vi "Sistema de ventilación_V4.vi"() -> ()   [LabVIEW 2023]
uses:
  <vilib>/MakerHub/LINX/Public/Peripherals/Analog/Analog Read 1 Chan.vi
  <vilib>/MakerHub/LINX/Public/Peripherals/Digital/Digital Write 1 Chan.vi
  <vilib>/MakerHub/LINX/Public/Peripherals/Analog/Analog Read N Chans.vi
  <vilib>/MakerHub/LINX/Public/Peripherals/Digital/Digital Write N Chans.vi
  <vilib>/MakerHub/LINX/Private/Local IO/LinxAnalogRead.vi
  <vilib>/MakerHub/LINX/Public/Utilities/Check Channel.vi
  <vilib>/MakerHub/LINX/Private/Local IO/LinxDigitalWrite.vi
  <vilib>/MakerHub/LINX/Public/Utilities/Open Serial.vi
  <vilib>/MakerHub/LINX/Public/Sensors/Motion/Servo/Servo Open One Channel.vi
  <vilib>/MakerHub/LINX/Public/Peripherals/Analog/Analog Write 1 Chan.vi
  <vilib>/MakerHub/LINX/Private/Utilties/Generate Error.vi
  <vilib>/MakerHub/LINX/Public/Sensors/Motion/Servo/Servo Set Pulse Width One Channel.vi
  <vilib>/MakerHub/LINX/Public/Sensors/Motion/Servo/Servo Close One Channel.vi
  <vilib>/MakerHub/LINX/LMH-LINX.lvlib
  <vilib>/MakerHub/LINX/Public/Sensors/Motion/Servo/Servo.lvlib
panel:
  in  "Temp":dbl(knob) scale=-20.0..100.0
  in  "Aire":dbl(knob) scale=0.0..1000.0
  out "?":bool
  out "?":bool
  out "?":bool
  out "?":bool
  in  "?":bool
  out "Serevo Aire Angulo":string
  out "Serevo Temp Angulo":string
  in  "Serial Port":refnum<visa-resource-name>
  out "?":bool
  out "?":bool
  out "?":bool
  out "?":bool
  out "?":bool
  out "?":bool
  out "?":bool
  out "?":bool
  out "?":bool
  out "?":bool
  out "?":bool
  out "?":bool
  out "?":bool
  out "?":bool
  out "?":bool
  out "?":bool
  out "?":bool
  out "?":bool
  in  "?":bool
  out "Filtro de Calor":bool
  out "Filtro de Aire":bool
  out "Ppm del aire":dbl(knob) scale=0.0..1800.0
  out "Temperatura":dbl(slide) scale=0.0..60.0
  out "t [sec]":dbl
  out "Iteration No":i32
  in  "?":bool
  out "VI is running?":bool caption="ON/OFF"
  # "SISTEMA DE VENTILACIÓN DE DOBLE FLUJO"
  # "Temperatura"
  # "Entrada"
  # "Calidad del aire"
  # "Salida"
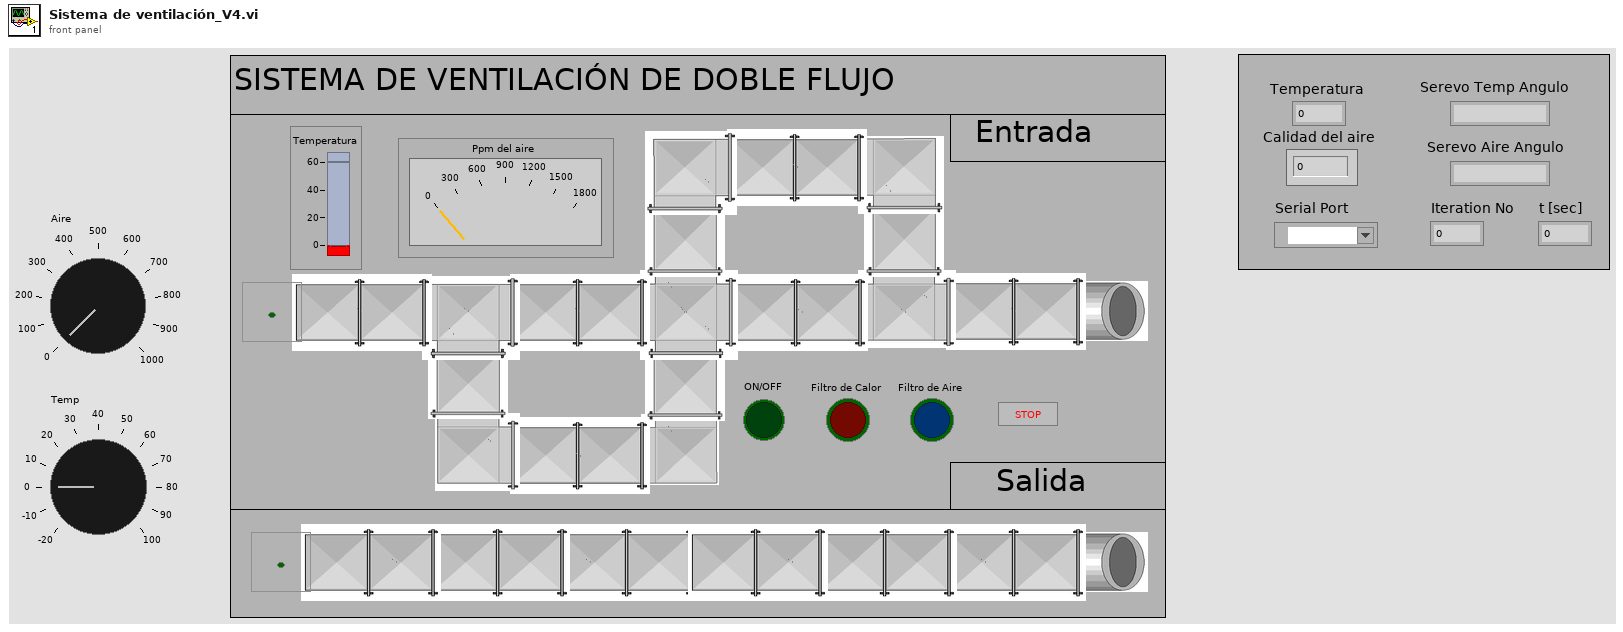
[diagram p1: front panel]
types:
  T1 = typedef "LMH-LINX.lvlib/LINX Ref.ctl" = cluster{"IO":T2, "Interface":T3, "LINX Device Config":T4}
  T2 = typedef "LMH-LINX.lvlib/Platform.ctl" = enum16{"Remote", "Local"}
  T3 = typedef "LMH-LINX.lvlib/Interface.ctl" = enum16{"Serial", "TCP"}
  T4 = typedef "LMH-LINX.lvlib/Device.lvlib/LINX Device Config.ctl" = cluster{"Interface":T3, "COM Port":refnum<visa-resource-name>, "TCP Configuration":T5, "Device Family":u8, "Device ID":u8, "Device Name":string, "TCP Ref":refnum<k5>, "Channels":T6}
  T5 = typedef "LMH-LINX.lvlib/Device.lvlib/TCP Config.ctl" = cluster{"IP Address":string, "Port":u16}
  T6 = typedef "LMH-LINX.lvlib/Channels.ctl" = cluster{"DI":u8[], "DO":u8[], "AI":u8[], "AO":u8[], "PWM":u8[], "QE":u8[], "UART":u8[], "I2C 2":u8[], "SPI":u8[], "CAN":u8[], "Servo":u8[], "AI Ref (V)":dbl, "AI Resolution (Bits)":u8, "AO Ref (V)":dbl, "AO Resolution (Bits)":u8}
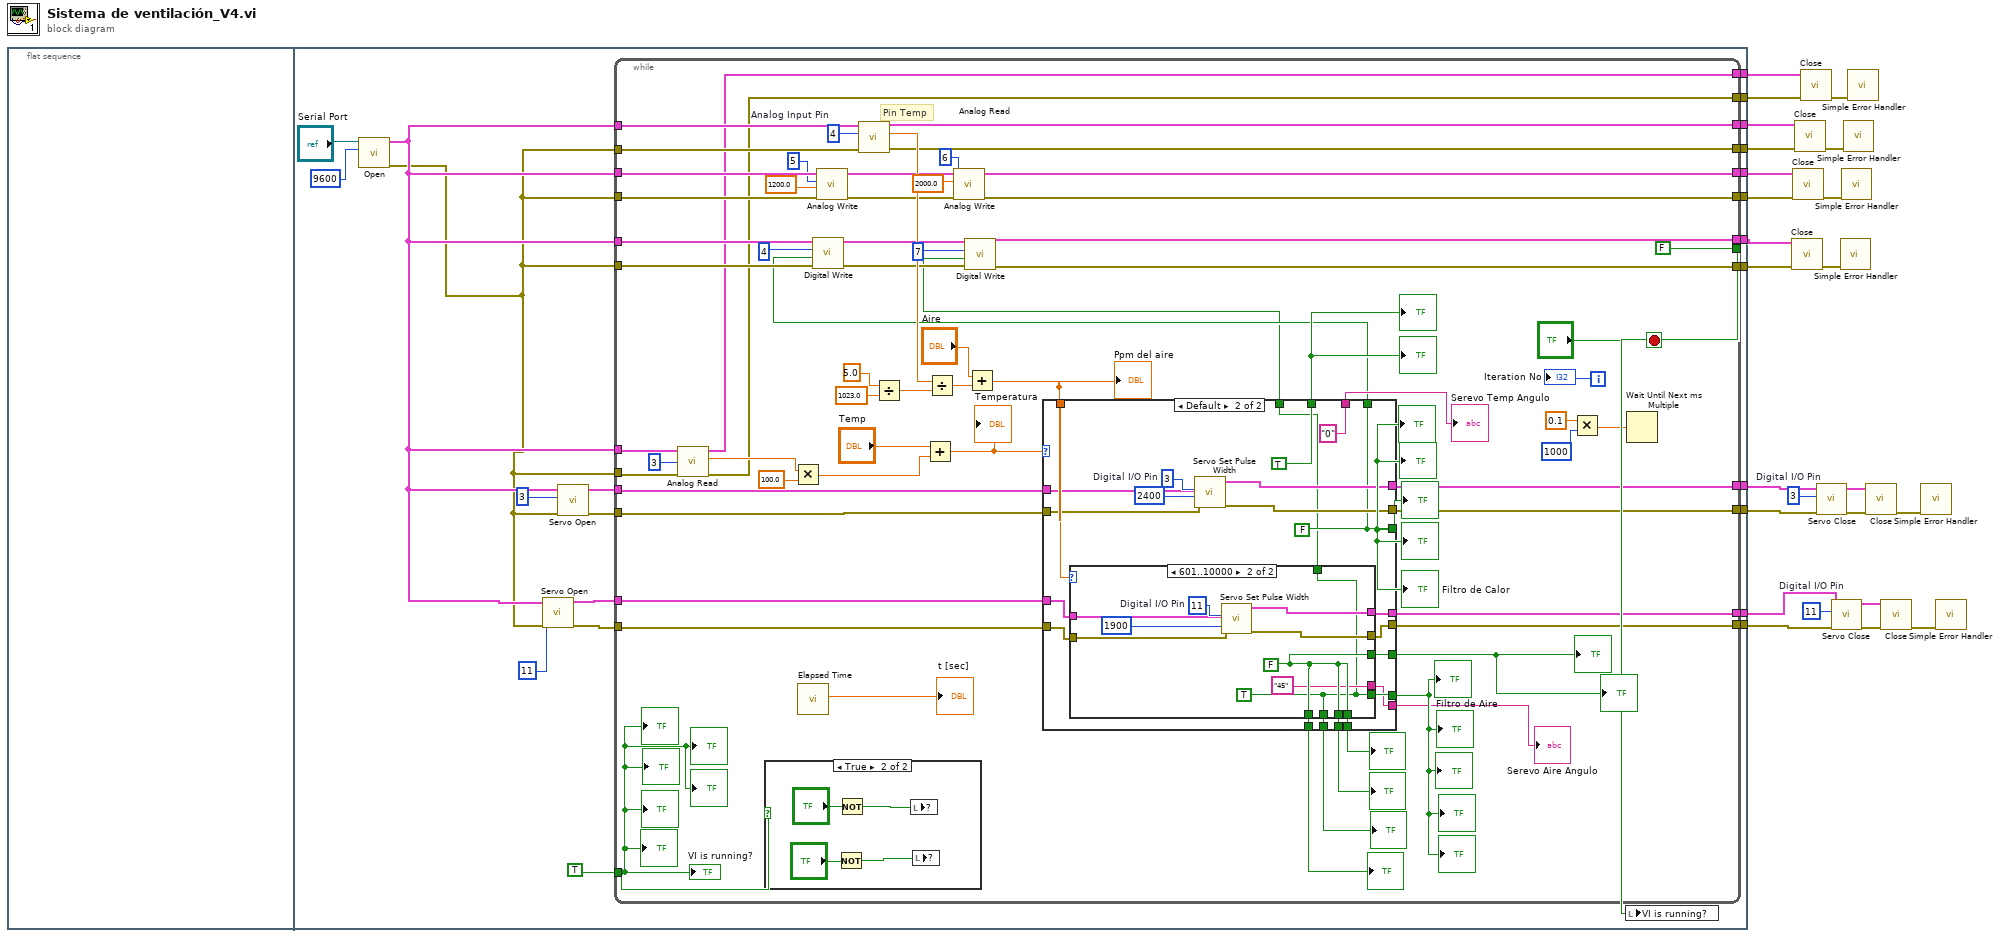
[diagram p0: block diagram]
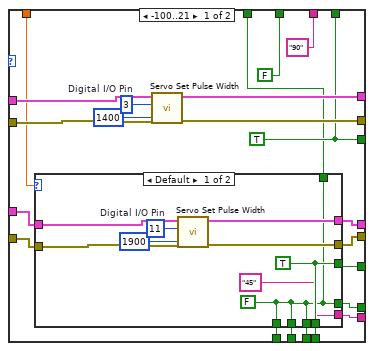
[diagram p2: hidden frame]
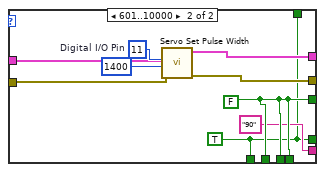
[diagram p3: hidden frame]
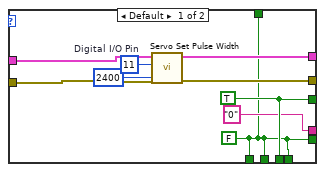
[diagram p4: hidden frame]
diagram:
  w7 = 11  # Digital I/O Pin
  w13 = 3  # Digital I/O Pin
  n1 = flat-sequence {
    tunnel: [w45] -> w24
    tunnel: [w43] -> w22
    tunnel: [w42] -> w20
    tunnel: [w41] -> w19
    tunnel: [w40] -> w17
    tunnel: [w39] -> w16
    tunnel: [w38] -> w1
    tunnel: [w37] -> w14
    tunnel: [w34] -> w9
    tunnel: [w33] -> w8
    tunnel: [w32] -> w3
    tunnel: [w31] -> w2
    frame #0 {
    }
    frame #1 {
      n2 = call-poly <vilib>:"Open.vi"("Baud Rate Override"=u32 9600, "Serial Port"="Serial Port") -> ("Error Out"=w27:errorcluster, "LINX Resource"=w29:T1)  [unwired: 7 in, 1 out]
      n3 = call-poly <vilib>:"Servo Open.vi"("Error In"=w27, "Servo Channel"=u8 11, "LINX Resource"=w29) -> ("Error Out"=w26:errorcluster, "LINX Resource"=w28:T1)  [unwired: 7 in]
      n4 = call-poly <vilib>:"Servo Open.vi"("Error In"=w27, "Servo Channel"=u8 3, "LINX Resource"=w29) -> ("Error Out"=w35:errorcluster, "LINX Resource"=w36:T1)  [unwired: 7 in]
      n5 = while {
        tunnel: [FALSE] -> w47
        tunnel: TRUE -> [w90]
        tunnel: w29 -> [w53]
        tunnel: [w55] -> w45
        tunnel: w27 -> [w52]
        tunnel: w29 -> [w109]
        tunnel: [w54] -> w43
        tunnel: w27 -> [w104]
        tunnel: [w102] -> w42
        tunnel: [w101] -> w41
        tunnel: w27 -> [w100]
        tunnel: w29 -> [w99]
        tunnel: [w92] -> w40
        tunnel: [w91] -> w39
        tunnel: w27 -> [w89]
        tunnel: w29 -> [w88]
        tunnel: [w83] -> w38
        tunnel: [w82] -> w37
        tunnel: w36 -> [w81]
        tunnel: w35 -> [w80]
        tunnel: [w79] -> w34
        tunnel: [w78] -> w33
        tunnel: w28 -> [w72]
        tunnel: w26 -> [w71]
        tunnel: [w70] -> w32
        tunnel: [w69] -> w31
        i -> [w111]
        stop <- "?" stop-if-true
        w103 = 4  # Analog Input Pin
        # "Pin Temp"
        n6 = call-poly <vilib>:"Analog Read.vi"("Error In"=w52, "Analog Channel"=u8 3, "LINX Resource"=w53) -> ("Error Out"=w54:errorcluster, "Voltage"=w57:dbl, "LINX Resource"=w55:T1)  [unwired: 5 in, 1 out]
        n7 = case shown="True" w90 {
          frame False {
          }
          frame True {
            n8 = Not(x="?") -> (.not. x?=w197:bool)
            n9 = Not(x="?") -> (.not. x?=w199:bool)
            n10 = local write item#8(w199) -> ()
            n11 = local write item#30(w197) -> ()
          }
        }
        n12 = Multiply(x=w57, y=100.0 ("x")) -> (x*y=w56:dbl)
        n13 = call "Elapsed Time"() -> ("Elapsed Time (s)"=→"t [sec]":dbl)  [unwired: 12 in, 7 out]
        n14 = call-poly <vilib>:"Analog Write.vi"("Error In"=w100, "AO Value"=1200.0, "AO Channel"=5, "LINX Resource"=w99) -> ("Error Out"=w93:errorcluster, "LINX Resource"=w94:T1)  [unwired: 6 in]
        n15 = call-poly <vilib>:"Analog Read.vi"("Error In"=w104, "Analog Channel"=w103, "LINX Resource"=w109) -> ("Error Out"=w101:errorcluster, "Voltage"=w106:dbl, "LINX Resource"=w102:T1)  [unwired: 5 in, 1 out]
        n16 = Divide(x=5.0, y=1023.0) -> (x/y=w105:dbl)
        n17 = Add(x="Temp", y=w56) -> (x+y=w74:dbl)
        "Temperatura" <- w74
        n18 = Divide(x=w106, y=w105) -> (x/y=w76:dbl)
        n19 = call-poly <vilib>:"Analog Write.vi"("Error In"=w93, "AO Value"=2000.0, "AO Channel"=6, "LINX Resource"=w94) -> ("Error Out"=w92:errorcluster, "LINX Resource"=w91:T1)  [unwired: 6 in]
        n20 = Add(x="Aire", y=w76) -> (x+y=w68:dbl)
        "Ppm del aire" <- w68
        n21 = case shown="Default" w74 {
          tunnel: w81 -> [w136 w176]
          tunnel: w80 -> [w135 w175]
          tunnel: [w134 w174] -> w79
          tunnel: [w133 w173] -> w78
          tunnel: [w118 w158] -> w73
          tunnel: [FALSE TRUE] -> w51
          tunnel: w72 -> [w128 w166]
          tunnel: w71 -> [w127 w165]
          tunnel: [w125 w167] -> w70
          tunnel: [w126 w168] -> w69
          tunnel: w68 -> [w129 w169]
          tunnel: [w131 w171] -> w67
          tunnel: [w130 w170] -> w66
          tunnel: [w124 w164] -> w65
          tunnel: [w121 w163] -> w64
          tunnel: [w122 w162] -> w63
          tunnel: [w123 w161] -> w62
          tunnel: ["90" ("Serevo Temp Angulo") "0" ("Serevo Temp Angulo")] -> w61
          tunnel: [w119 w159] -> w60
          tunnel: [w118 w158] -> w50
          tunnel: [w117 w157] -> w49
          frame -100..21 {
            w118 = TRUE
            w138 = 3  # Digital I/O Pin
            n22 = case shown="Default" w129 {
              tunnel: w128 -> [w145 w154]
              tunnel: w127 -> [w144 w153]
              tunnel: [w143 w152] -> w126
              tunnel: [w142 w151] -> w125
              tunnel: [w141 w150] -> w131
              tunnel: [w139 w148] -> w130
              tunnel: [w141 w150] -> w124
              tunnel: [w139 w148] -> w123
              tunnel: [w139 w150] -> w122
              tunnel: [w139 w150] -> w121
              tunnel: ["45" ("Serevo Aire Angulo") "90" ("Serevo Aire Angulo")] -> w119
              tunnel: [w139 w148] -> w117
              frame Default {
                w139 = FALSE
                w141 = TRUE
                w147 = 11  # Digital I/O Pin
                n23 = call-poly <vilib>:"Servo Set Pulse Width.vi"("Error In"=w144, "Pulse Width (uS)"=u16 1900, "Servo Channel"=w147, "LINX Resource"=w145) -> ("Error Out"=w142:errorcluster, "LINX Resource"=w143:T1)  [unwired: 6 in]
              }
              frame 601..10000 {
                w150 = FALSE
                w148 = TRUE
                w156 = 11  # Digital I/O Pin
                n24 = call-poly <vilib>:"Servo Set Pulse Width.vi"("Error In"=w153, "Pulse Width (uS)"=u16 1400, "Servo Channel"=w156, "LINX Resource"=w154) -> ("Error Out"=w151:errorcluster, "LINX Resource"=w152:T1)  [unwired: 6 in]
              }
            }
            n25 = call-poly <vilib>:"Servo Set Pulse Width.vi"("Error In"=w135, "Pulse Width (uS)"=u16 1400, "Servo Channel"=w138, "LINX Resource"=w136) -> ("Error Out"=w133:errorcluster, "LINX Resource"=w134:T1)  [unwired: 6 in]
          }
          frame Default {
            w158 = FALSE
            w178 = 3  # Digital I/O Pin
            n26 = case shown="601..10000" w169 {
              tunnel: w166 -> [w185 w195]
              tunnel: w165 -> [w184 w194]
              tunnel: [w183 w193] -> w168
              tunnel: [w182 w192] -> w167
              tunnel: [w181 w191] -> w171
              tunnel: [w179 w189] -> w170
              tunnel: [w179 w191] -> w164
              tunnel: [w181 w191] -> w163
              tunnel: [w179 w189] -> w162
              tunnel: [w179 w191] -> w161
              tunnel: ["0" ("Serevo Aire Angulo") "45" ("Serevo Aire Angulo")] -> w159
              tunnel: [w179 w189] -> w157
              frame Default {
                w179 = FALSE
                w181 = TRUE
                w187 = 11  # Digital I/O Pin
                n27 = call-poly <vilib>:"Servo Set Pulse Width.vi"("Error In"=w184, "Pulse Width (uS)"=u16 2400, "Servo Channel"=w187, "LINX Resource"=w185) -> ("Error Out"=w182:errorcluster, "LINX Resource"=w183:T1)  [unwired: 6 in]
              }
              frame 601..10000 {
                w191 = FALSE
                w189 = TRUE
                w196 = 11  # Digital I/O Pin
                n28 = call-poly <vilib>:"Servo Set Pulse Width.vi"("Error In"=w194, "Pulse Width (uS)"=u16 1900, "Servo Channel"=w196, "LINX Resource"=w195) -> ("Error Out"=w192:errorcluster, "LINX Resource"=w193:T1)  [unwired: 6 in]
              }
            }
            n29 = call-poly <vilib>:"Servo Set Pulse Width.vi"("Error In"=w175, "Pulse Width (uS)"=u16 2400, "Servo Channel"=w178, "LINX Resource"=w176) -> ("Error Out"=w173:errorcluster, "LINX Resource"=w174:T1)  [unwired: 6 in]
          }
        }
        "?" <- w63
        "?" <- w64
        "?" <- w62
        "?" <- w65
        "Serevo Temp Angulo" <- w61
        "Serevo Aire Angulo" <- w60
        "?" <- w73
        "?" <- w73
        "?" <- w73
        "?" <- w73
        "Filtro de Calor" <- w73
        "?" <- w51
        "?" <- w51
        "Filtro de Aire" <- w66
        "?" <- w66
        "?" <- w66
        "?" <- w66
        "?" <- w66
        "?" <- w67
        "?" <- w67
        n30 = call-poly <vilib>:"Digital Write.vi"("Error In"=w89, "Output Value"=w50, "DO Channel"=4, "LINX Resource"=w88) -> ("Error Out"=w84:errorcluster, "LINX Resource"=w85:T1)  [unwired: 6 in]
        n31 = call-poly <vilib>:"Digital Write.vi"("Error In"=w84, "Output Value"=w49, "DO Channel"=7, "LINX Resource"=w85) -> ("Error Out"=w82:errorcluster, "LINX Resource"=w83:T1)  [unwired: 6 in]
        n32 = Multiply(x=0.1, y=1000) -> (x*y=w114:dbl)
        n33 = Wait Until Next ms Multiple(millisecond multiple=w114) -> ()  [unwired: 1 out]
        "VI is running?" <- w90
        "Iteration No" <- w111
        "?" <- w90
        "?" <- w90
        "?" <- w90
        "?" <- w90
        "?" <- w90
        "?" <- w90
      }
      n34 = local write "VI is running?"(w47) -> ()
    }
  }
  n35 = call <vilib>:"Close.vi"("Error In"=w14, "LINX Resource"=w1) -> ("Error Out"=w15:errorcluster)  [unwired: 9 in]
  n36 = call <vilib>:"Close.vi"("Error In"=w17, "LINX Resource"=w16) -> ("Error Out"=w18:errorcluster)  [unwired: 9 in]
  n37 = call <vilib>:"Close.vi"("Error In"=w19, "LINX Resource"=w20) -> ("Error Out"=w21:errorcluster)  [unwired: 9 in]
  n38 = call <vilib>:"Close.vi"("Error In"=w22, "LINX Resource"=w24) -> ("Error Out"=w23:errorcluster)  [unwired: 9 in]
  n39 = call-poly <vilib>:"Servo Close.vi"("Error In"=w8, "Servo Channel"=w13, "LINX Resource"=w9) -> ("Error Out"=w11:errorcluster, "LINX Resource"=w12:T1)  [unwired: 7 in]
  n40 = call-poly <vilib>:"Servo Close.vi"("Error In"=w3, "Servo Channel"=w7, "LINX Resource"=w2) -> ("Error Out"=w5:errorcluster, "LINX Resource"=w6:T1)  [unwired: 7 in]
  n41 = call <vilib>:"Simple Error Handler.vi"("error in (no error)"=w15) -> ()  [unwired: 4 in, 5 out]
  n42 = call <vilib>:"Simple Error Handler.vi"("error in (no error)"=w18) -> ()  [unwired: 4 in, 5 out]
  n43 = call <vilib>:"Simple Error Handler.vi"("error in (no error)"=w21) -> ()  [unwired: 4 in, 5 out]
  n44 = call <vilib>:"Simple Error Handler.vi"("error in (no error)"=w23) -> ()  [unwired: 4 in, 5 out]
  n45 = call <vilib>:"Close.vi"("Error In"=w11, "LINX Resource"=w12) -> ("Error Out"=w10:errorcluster)  [unwired: 9 in]
  n46 = call <vilib>:"Close.vi"("Error In"=w5, "LINX Resource"=w6) -> ("Error Out"=w4:errorcluster)  [unwired: 9 in]
  n47 = call <vilib>:"Simple Error Handler.vi"("error in (no error)"=w10) -> ()  [unwired: 4 in, 5 out]
  n48 = call <vilib>:"Simple Error Handler.vi"("error in (no error)"=w4) -> ()  [unwired: 4 in, 5 out]
